vi "State5-Back In.vi"(11 "Numeric":dbl) -> (1 "Cluster":T2, 2 "Front/Back 2":enum16{"Forward", "Backward", "Stop"}(ring), 3 "Left/Right":enum16{"Left", "Right", "Stop"}(ring), 4 "Enum":T1, 5 "Left/Right Speed":u32)   [LabVIEW 2014]
uses:
  FPGA Bitfiles/Parking States Indicators.ctl
  FPGA Bitfiles/Parking States.ctl
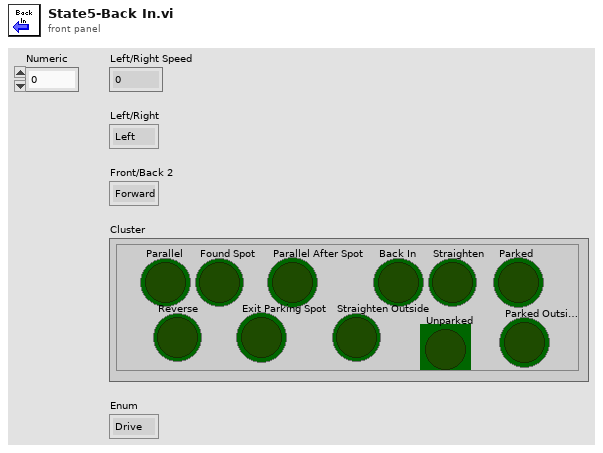
[diagram p1: front panel]
types:
  T1 = typedef "Parking States.ctl" = enum16{"Drive", "Parallel", "Found Spot", "Parallel After Spot", "Back In", "Straighten", "Parked", "Reverse", "Exit Parking Spot", "Straighten Outside", "Unparked", "Parked Outside"}
  T2 = typedef "Parking States Indicators.ctl" = cluster{"Parallel":bool, "Found Spot":bool, "Parallel After Spot":bool, "Back In":bool, "Straighten":bool, "Parked":bool, "Reverse":bool, "Exit Parking Spot":bool, "Straighten Outside":bool, "Unparked":bool, "Parked Outside":bool}
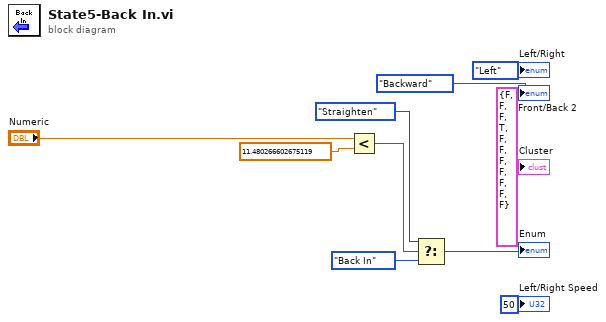
[diagram p0: block diagram]
diagram:
  n1 = Less?(x="Numeric", y=11.480266602675119 ("Reverse threshold")) -> (x < y?=w4:bool)
  n2 = Select(t=Parking_States."Straighten", s=w4, f=Parking_States."Back In") -> (s? t:f=→"Enum":T1)
  "Cluster" <- T2 {"Parallel"=FALSE, "Found Spot"=FALSE, "Parallel After Spot"=FALSE, "Back In"=TRUE, "Straighten"=FALSE, "Parked"=FALSE, "Reverse"=FALSE, "Exit Parking Spot"=FALSE, "Straighten Outside"=FALSE, "Unparked"=FALSE, "Parked Outside"=FALSE} ("Cluster")
  "Front/Back 2" <- enum16{"Forward", "Backward", "Stop"}."Backward" ("Front/Back 2")
  "Left/Right" <- enum16{"Left", "Right", "Stop"}."Left" ("Left/Right")
  "Left/Right Speed" <- u32 50 ("Left/Right Speed")
